vi "Set Channel Sampling Period.vi"(8 "error in (no error)":errorcluster, 9 "Sampling Period":u16(ring)=1 items=["1ms"=1, "2ms"=2, "5ms"=5, "10ms"=10, "20ms"=20, "50ms"=50, "100ms"=100], 10 "Channel":u16(ring) items=["A1"=0, "A2"=1, "A3"=2, "A4"=3, "A5"=4, "A6"=5, "A7"=6, "A8"=7, "A9"=8, "A10"=9, "K1"=200, "K2"=201, "K3"=202, "K4"=203, "FA1"=204, "FA2"=205, "FA3"=206, "FA4"=207], 11 "VISA resource name":refnum<visa-resource-name>) -> (0 "error out":errorcluster, 3 "VISA resource name out":refnum<visa-resource-name>)   [LabVIEW 2017, in "Sefram DAS220.lvlib"]
doc: "Define the channel sampling period from 1ms to 100ms.\n<B>For Pt100/Pt1000</B> the sampling period is twice as much."
uses:
  <instrlib>/Sefram DAS220/Sefram DAS220.lvlib
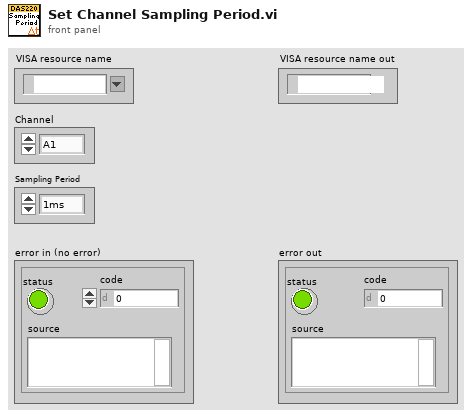
[diagram p1: front panel]
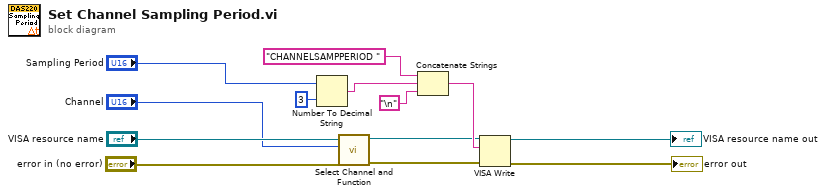
[diagram p0: block diagram]
diagram:
  n1 = Number To Decimal String(number="Sampling Period", width (-)=i16 3) -> (decimal integer string=w6:string)
  n2 = call <instrlib>:"Select Channel and Function.vi"("error in (no error)"="error in (no error)", "Channel"="Channel", "VISA resource name"="VISA resource name") -> ("error out"=w4:errorcluster, "VISA resource name out"=w2:refnum<visa-resource-name>)  [unwired: 7 in]
  n3 = Concatenate Strings("CHANNELSAMPPERIOD " ("string"), w6, "\n") -> (w12:string)
  n4 = VISA Write(VISA resource name=w2, write buffer=w12, error in (no error)=w4) -> (VISA resource name out=→"VISA resource name out":refnum<visa-resource-name>, error out=→"error out":errorcluster)  [unwired: 1 out]
